vi "Close Drive.vi"(8 "error in":errorcluster) -> (0 "error out":errorcluster)   [LabVIEW 2018]
uses:
  TypeDefs/typedef_enum_Refnums.ctl
  <vilib>/Rock Robotics/WPI/Utilities/WPI_GetSetVariantRefNum.vi
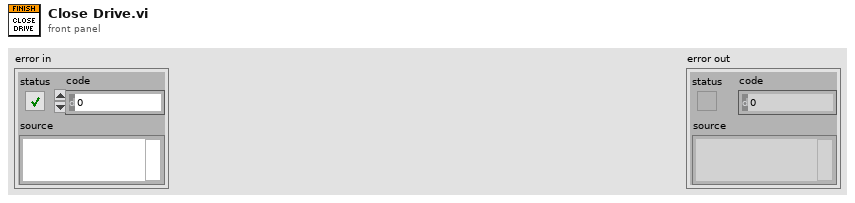
[diagram p1: front panel]
types:
  T1 = typedef "typedef_enum_Refnums.ctl" = enum16{"Ball_Encoder", "Ball_Motor", "Camera", "Linefollow_3", "Linefollow_2", "Linefollow_1", "Gyro", "Hatch_Solenoid", "Climb_Back_Solenoid", "Arm_Encoder", "Arm_Motor", "Lift_Encoder", "Drive", "Drive_Motor_R", "Drive_Motor_L", "Drive_Encoder_R", "Drive_Encoder_L", "Joy_R", "Joy_L", "Wrist_Motor", "Wrist_Encoder", "Climb Upper Limit", "Climb Lower Limit ", "Climb_Front_Motor"}
  T2 = typedef "WPI_RobotDriveDevRef.ctl" = cluster{"DevStatus":errorcluster, "Motors[]":T3[], "Square Inputs":bool, "Max Output":dbl}
  T3 = typedef "WPI_MotorControlDeviceRef.ctl" = cluster{"DeviceStatus":errorcluster, "Type":T4, "PWM":cluster{"PWM Channel":T5, "DeadBand":T6}, "CAN":cluster{"Device Number":u8, "SetOutput VI Ref":variant, "GetOutput VI Ref":variant, "Enable VI Ref":variant, "Disable VI Ref":variant, "Data":variant}, "Invert":bool, "DIO PWM":cluster{"PWM \"Enable\" Channel":T5, "DIOChannel":T7, "PWM Rate":dbl}}
  T4 = typedef "WPI_MotorControlType.ctl" = enum16{"PWM", "CAN", "DIO PWM"}
  T5 = typedef "FPGA_DIOPWMChannel.ctl" = enum8{"PWM 0", "PWM 1", "PWM 2", "PWM 3", "PWM 4", "PWM 5", "PWM 6", "PWM 7", "PWM 8", "PWM 9", "PWM MXP 0", "PWM MXP 1", "PWM MXP 2", "PWM MXP 3", "PWM MXP 4", "PWM MXP 5", "PWM MXP 6", "PWM MXP 7", "PWM MXP 8", "PWM MXP 9", "Invalid"}
  T6 = typedef "WPI_PWMDeadband.ctl" = cluster{"Name":string, "maxPositivePwm":i32, "minPositivePwm":i32, "centerPwm":i32, "maxNegativePwm":i32, "minNegativePwm":i32, "angularRange":u16}
  T7 = typedef "FPGA_DIOChannel.ctl" = enum8{"DIO 0", "DIO 1", "DIO 2", "DIO 3", "DIO 4", "DIO 5", "DIO 6", "DIO 7", "DIO 8", "DIO 9", "DIO MXP 0", "DIO MXP 1", "DIO MXP 2", "DIO MXP 3", "DIO MXP 4", "DIO MXP 5", "DIO MXP 6", "DIO MXP 7", "DIO MXP 8", "DIO MXP 9", "DIO MXP 10", "DIO MXP 11", "DIO MXP 12", "DIO MXP 13", "DIO MXP 14", "DIO MXP 15", "SPI Port CS1", "SPI Port CS2", "SPI Port CS3", "SPI Port MISO", "SPI Port MOSI", "Invalid"}
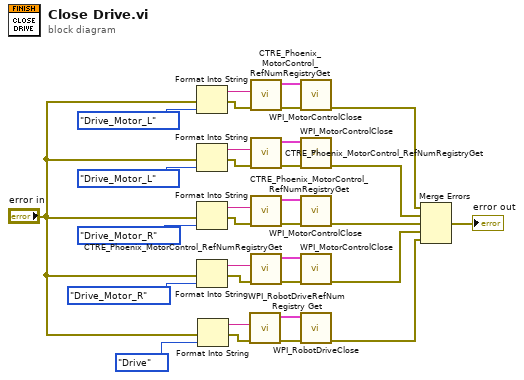
[diagram p0: block diagram]
diagram:
  n1 = Format Into String(error in="error in", typedef_enum_Refnums."Drive_Motor_L" ("RefNums")) -> (resulting string=w23:string, error out=w13:errorcluster)  [unwired: 2 in]
  n2 = Format Into String(error in="error in", typedef_enum_Refnums."Drive_Motor_L" ("RefNums")) -> (resulting string=w14:string, error out=w21:errorcluster)  [unwired: 2 in]
  n3 = Format Into String(error in="error in", typedef_enum_Refnums."Drive_Motor_R" ("RefNums")) -> (resulting string=w17:string, error out=w16:errorcluster)  [unwired: 2 in]
  n4 = Format Into String(error in="error in", typedef_enum_Refnums."Drive_Motor_R" ("RefNums")) -> (resulting string=w18:string, error out=w15:errorcluster)  [unwired: 2 in]
  n5 = Format Into String(error in="error in", typedef_enum_Refnums."Drive" ("RefNums")) -> (resulting string=w1:string, error out=w3:errorcluster)  [unwired: 2 in]
  n6 = call <vilib>:"WPI_RobotDriveRefNum Registry Get.vi"("error in (no error)"=w3, "refnum name"=w1) -> ("error out"=w12:errorcluster, "RobotDriveDevRef"=w11:T2)  [unwired: 8 in]
  n7 = call <vilib>:"CTRE_Phoenix_MotorControl_RefNumRegistryGet.vi"("error in (no error)"=w13, "refnum name"=w23) -> ("error out"=w30:errorcluster, "PhoenixMotorControlDevRef"=w29:T3)  [unwired: 8 in]
  n8 = call <vilib>:"CTRE_Phoenix_MotorControl_RefNumRegistryGet.vi"("error in (no error)"=w21, "refnum name"=w14) -> ("error out"=w32:errorcluster, "PhoenixMotorControlDevRef"=w31:T3)  [unwired: 8 in]
  n9 = call <vilib>:"CTRE_Phoenix_MotorControl_RefNumRegistryGet.vi"("error in (no error)"=w16, "refnum name"=w17) -> ("error out"=w27:errorcluster, "PhoenixMotorControlDevRef"=w28:T3)  [unwired: 8 in]
  n10 = call <vilib>:"CTRE_Phoenix_MotorControl_RefNumRegistryGet.vi"("error in (no error)"=w15, "refnum name"=w18) -> ("error out"=w25:errorcluster, "PhoenixMotorControlDevRef"=w26:T3)  [unwired: 8 in]
  n11 = call <vilib>:"WPI_MotorControlClose.vi"("error in"=w30, "MotorControlDevRef"=w29) -> ("error out"=w6:errorcluster)  [unwired: 9 in]
  n12 = call <vilib>:"WPI_MotorControlClose.vi"("error in"=w32, "MotorControlDevRef"=w31) -> ("error out"=w7:errorcluster)  [unwired: 9 in]
  n13 = call <vilib>:"WPI_MotorControlClose.vi"("error in"=w27, "MotorControlDevRef"=w28) -> ("error out"=w8:errorcluster)  [unwired: 9 in]
  n14 = call <vilib>:"WPI_MotorControlClose.vi"("error in"=w25, "MotorControlDevRef"=w26) -> ("error out"=w9:errorcluster)  [unwired: 9 in]
  n15 = call <vilib>:"WPI_RobotDriveClose.vi"("error in (no error)"=w12, "RobotDriveDevRef"=w11) -> ("error out"=w10:errorcluster)  [unwired: 9 in]
  n16 = Merge Errors(w6, w7, w8, w9, w10) -> (→"error out":errorcluster)
